vi "Configure Sine.vi"(0 "template configuration":refnum<class "SV Signal.lvclass">, 5 "frequency (Hz)":dbl=1000.0, 7 "amplitude":dbl=1.0, 9 "phase (deg)":dbl, 11 "error in (no error)":errorcluster) -> (4 "signal configuration":refnum<class "SV Sinusoid.lvclass">, 15 "error out":errorcluster)   [LabVIEW 2017, in "SV Sinusoid.lvclass"]
doc: "Configures a user-defined test signal. Wire the outputs to SV Signal (waveform) VI to generate the test signal, or wire to SV Signal Property Node to configure additional parameters before wiring to the SV Signal (waveform) VI."
uses:
  <vilib>/addons/_NISVFA/_Generation/Signal Generation/SV Sinusoid/SV Sinusoid.lvclass
  C:/Program Files (x86)/National Instruments/LabVIEW 2017/vi.lib/addons/_NISVFA/_Generation/Signal Generation/SV Function/SV Function.lvclass
  C:/Program Files (x86)/National Instruments/LabVIEW 2017/vi.lib/addons/_NISVFA/_Generation/Signal Generation/SV Signal/SV Signal.lvclass
  <vilib>/addons/_NISVFA/_Generation/Signal Generation/SV Signal/SV Signal.lvclass
  <vilib>/addons/_NISVFA/_Generation/Signal Generation/SV Signal/Write Measurement Duration.vi
  <vilib>/addons/_NISVFA/_Generation/Signal Generation/SV Signal/Write Sample Rate.vi
  <vilib>/addons/_NISVFA/_Generation/Signal Generation/SV Function/SV Function.lvclass
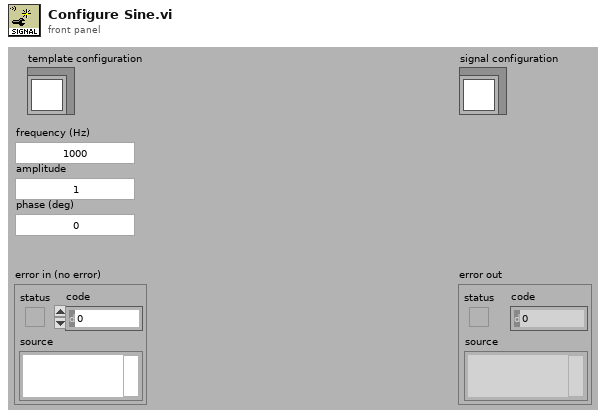
[diagram p1: front panel]
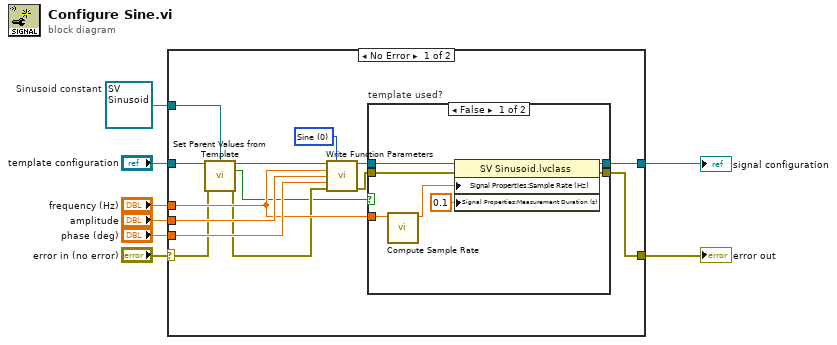
[diagram p0: block diagram]
diagram:
  w1 = refnum<class "SV Sinusoid.lvclass"> refnum  # Sinusoid constant
  n1 = case shown="No Error" "error in (no error)" {
    selector: "error in (no error)" -> [w11 w33]
    tunnel: [w17 w33] -> w7
    tunnel: [w18 w32] -> w3
    tunnel: "template configuration" -> [w14 _]
    tunnel: "frequency (Hz)" -> [w15 _]
    tunnel: "amplitude" -> [w22 _]
    tunnel: "phase (deg)" -> [w21 _]
    tunnel: w1 -> [w12 w32]
    frame No Error {
      w20 = u16 0 items=["Sine", "Triangle", "Square", "Sawtooth"] ("function type")
      n2 = call-dynamic "Set Parent Values from Template.vi"("template configuration"=w14, "signal configuration in"=w12, "error in (no error)"=w11) -> ("signal configuration out"=w13:refnum<class "SV Sinusoid.lvclass">, "template used?"=w9:bool, "error out"=w10:errorcluster)  [unwired: 10 in]
      n3 = call <vilib>:"Write Function Parameters.vi"("signal configuration"=w13, "function type"=w20, "frequency (Hz)"=w15, "amplitude"=w22, "phase (deg)"=w21, "error in (no error)"=w10) -> ("signal configuration"=w19:refnum<class "SV Sinusoid.lvclass">, "error out"=w16:errorcluster)  [unwired: 8 in]
      n4 = case "template used?" shown="False" w9 {
        tunnel: w19 -> [w29 w31]
        tunnel: [w28 w31] -> w18
        tunnel: [w27 w30] -> w17
        tunnel: w16 -> [w26 w30]
        tunnel: w15 -> [w25 _]
        frame False {
          n5 = call <vilib>:"Compute Sample Rate.vi"("maximum frequency [Hz]"=w25) -> ("sample rate [Hz]"=w24:dbl)  [unwired: 10 in]
          n6 = property class="SV Sinusoid.lvclass"(reference=w29, error in=w26, "Signal Properties:Sample Rate (Hz)"=w24, "Signal Properties:Measurement Duration (s)"=0.1 ("Measurement Cycles")) -> (reference out=w28:refnum<class "SV Sinusoid.lvclass">, error out=w27:errorcluster)
        }
        frame True {
        }
      }
    }
    frame Error {
    }
  }
  "error out" <- w7
  "signal configuration" <- w3
